vi "Draw Flatten Pixmap__jki_lib_picture -- VI Tester.vi"(10 "image data":T1, 11 "picture":picture) -> (3 "new picture":picture)   [LabVIEW 2011]
doc: "Draws a 1-, 4-, 8-bit pixmap, 24-bit RGB pixmap or a 32-bit ARGB pixmap into a picture. The transparency information in the 32-bit ARGB pixmap will be used to draw the pixmap over the existing picture.\n\n<B>Copyright © 2006 James Kring, Inc. All rights reserved.</B>\n\nAuthor: Philippe Guerit <<B>philippe.guerit@jameskring.com</B>>\n<alternate_email: <B>PJM_LabVIEW@yahoo.com</B>>\n\nThis library is provided \"AS IS\" , WITHOUT WARRANTIES OR \nCONDITIONS OF ANY KIND, either express or implied.\n\n<B>James Kring, Inc.</B> -- http://www.jameskring.com"
uses:
  <vilib>/picture/picture.llb/imagedata.ctl
panel:
  in  "Case Constant\n(See Context Help)":bool
  # "Copyright © 2006 James Kring, Inc. All rights reserved.\n\nAuthor: Philippe Guerit <philippe.guerit@jameskring.com>\n<alternate_email: PJM_LabVIEW@yahoo.com>\n\nThis library is provided \"AS IS\" , WITHOUT WARRANTIES OR \nCONDITIONS OF ANY KIND, either express or implied.\n\nJames Kring, Inc. -- http://www.jameskring.com"
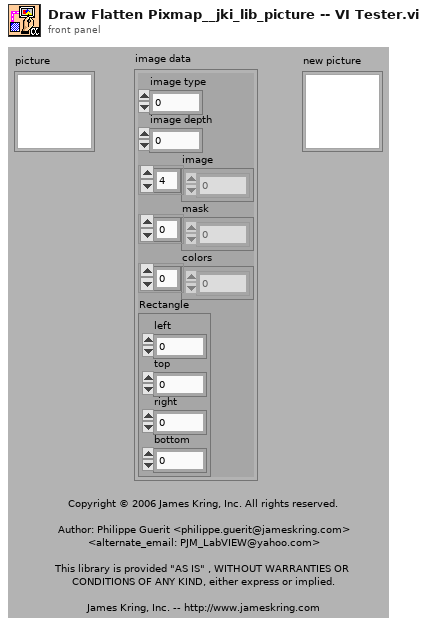
[diagram p1: front panel]
types:
  T1 = typedef "imagedata.ctl" = cluster{"image type":i32, "image depth":i32, "image":u8[], "mask":u8[], "colors":u32[], "Rectangle":cluster{"left":i16, "top":i16, "right":i16, "bottom":i16}}
  T2 = cluster{"left":i16, "top":i16, "right":i16, "bottom":i16}
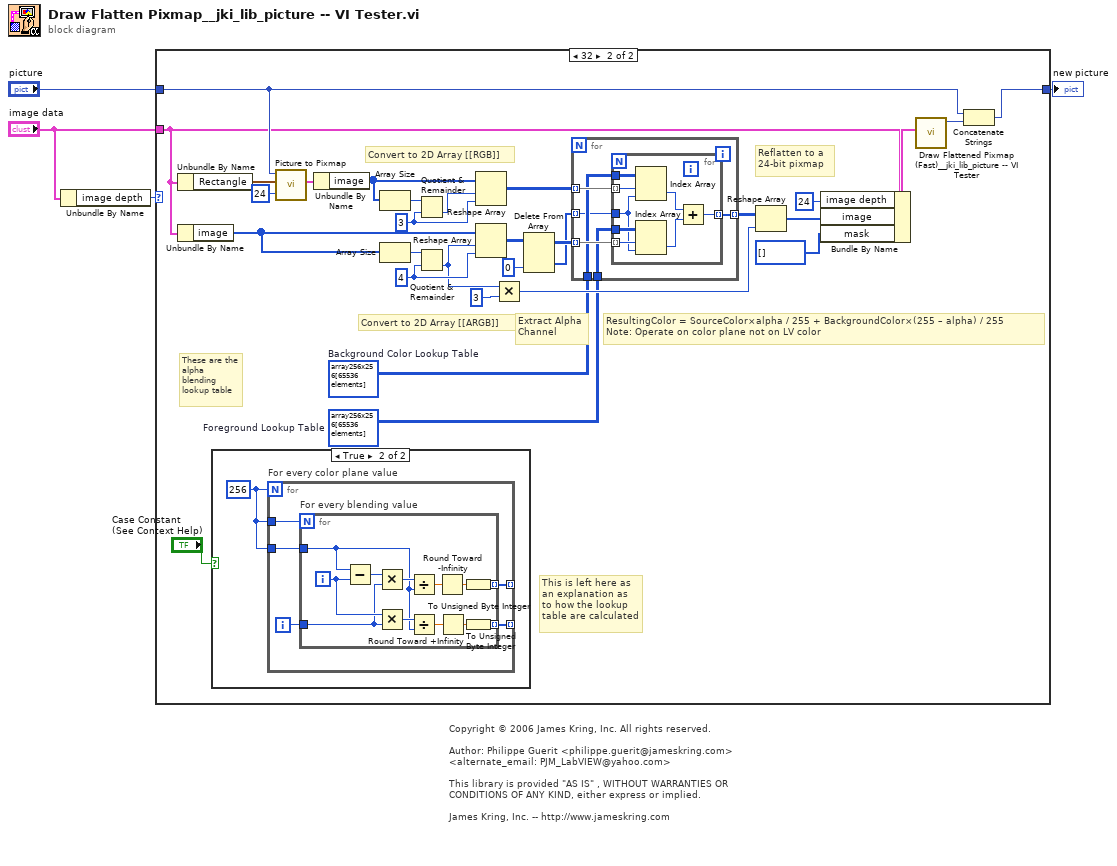
[diagram p0: block diagram]
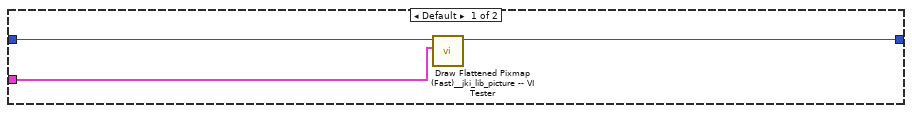
[diagram p2: hidden frame]
diagram:
  # "Copyright © 2006 James Kring, Inc. All rights reserved.\n\nAuthor: Philippe Guerit <philippe.guerit@jameskring.com>\n<alternate_email: PJM_LabVIEW@yahoo.com>\n\nThis library is provided \"AS IS\" , WITHOUT WARRANTIES OR \nCONDITIONS OF ANY KIND, either express or implied.\n\nJames Kring, Inc. -- http://www.jameskring.com"
  n1 = Unbundle By Name("image data") -> ("image depth"=w1:i32)
  n2 = case shown="32" w1 {
    tunnel: "image data" -> [w6 w12]
    tunnel: "picture" -> [w7 w18]
    tunnel: [w5 w19] -> w2
    frame Default {
      n3 = call "Draw Flattened Pixmap (Fast)__jki_lib_picture -- VI Tester.vi"("image data"=w6, "picture"=w7) -> ("new picture"=w5:picture)  [unwired: 7 in]
    }
    frame 32 {
      w9 = u8[][] array256x256[65536 elements]  # Foreground Lookup Table
      w10 = u8[][] array256x256[65536 elements]  # Background Color Lookup Table
      w30 = 3 ("y")
      w29 = 4 ("y")
      # "Reflatten to a 24-bit pixmap"
      # "Extract Alpha\nChannel"
      # "Convert to 2D Array [[ARGB]]"
      # "This is left here as an explanation as to how the lookup table are calculated"
      # "Convert to 2D Array [[RGB]]"
      # "These are the alpha blending lookup table"
      # "ResultingColor = SourceColor×alpha / 255 + BackgroundColor×(255 – alpha) / 255 \nNote: Operate on color plane not on LV color"
      n4 = Unbundle By Name(w12) -> ("Rectangle"=w37:T2)
      n5 = Unbundle By Name(w12) -> ("image"=w35:u8[])
      n6 = case shown="True" "Case Constant\n(See Context Help)" {
        frame False {
        }
        frame True {
          w38 = 256
          n7 = for "For every color plane value" {
            N: w38 -> [_]
            tunnel: w38 -> [w43]
            tunnel: w38 -> [w42]
            tunnel: [w40] -> _ mode=indexing
            tunnel: [w39] -> _ mode=indexing
            i -> [w41]
            n8 = for "For every blending value" {
              N: w43 -> [_]
              tunnel: w42 -> [w48]
              tunnel: w41 -> [w50]
              tunnel: [w53] -> w40 mode=indexing
              tunnel: [w46] -> w39 mode=indexing
              i -> [w52]
              n9 = Subtract(x=w48, y=w52) -> (x-y=w51:i32)
              n10 = Multiply(x=w51, y=w50) -> (x*y=w49:i32)
              n11 = Multiply(x=w52, y=w50) -> (x*y=w55:i32)
              n12 = Divide(x=w49, y=w48) -> (x/y=w47:dbl)
              n13 = Divide(x=w55, y=w48) -> (x/y=w54:dbl)
              n14 = Round Toward -Infinity(1:w47) -> (0:w45:dbl)
              n15 = Round Toward +Infinity(x=w54) -> (ceil(x): smallest int >= x=w44:dbl)
              n16 = To Unsigned Byte Integer(number=w45) -> (unsigned 8bit integer=w46:u8)
              n17 = To Unsigned Byte Integer(number=w44) -> (unsigned 8bit integer=w53:u8)
            }
          }
        }
      }
      n18 = call <vilib>:"Picture to Pixmap.vi"("depth"=24, "rect"=w37, "picture"=w18) -> ("image data"=w13:T1)  [unwired: 7 in, 1 out]
      n19 = Unbundle By Name(w13) -> ("image"=w31:u8[])
      n20 = Array Size(array=w31) -> (size(s)=w32:i32)
      n21 = Array Size(array=w35) -> (size(s)=w36:i32)
      n22 = Quotient & Remainder(x=w32, y=w30) -> (floor(x/y)=w22:i32)  [unwired: 1 out]
      n23 = Quotient & Remainder(x=w36, y=w29) -> (floor(x/y)=w26:i32)  [unwired: 1 out]
      n24 = Reshape Array(w31, w22, w30) -> (w14:u8[][])
      n25 = Reshape Array(w35, w26, w29) -> (w33:u8[][])
      n26 = Multiply(x=w26, y=3) -> (x*y=w25:i32)
      n27 = Delete From Array(array=w33, index (col)=0 ("dimension size")) -> (deleted portion=w15:u8[], array with subset deleted=w21:u8[][])  [unwired: 2 in]
      n28 = for {
        tunnel: w21 -> [w60] mode=indexing
        tunnel: w14 -> [w61] mode=indexing
        tunnel: w10 -> [w59]
        tunnel: w9 -> [w58]
        tunnel: [w56] -> w28 mode=indexing
        tunnel: w15 -> [w57] mode=indexing
        n29 = for {
          tunnel: w61 -> [w68] mode=indexing
          tunnel: w60 -> [w66] mode=indexing
          tunnel: w59 -> [w69]
          tunnel: w58 -> [w67]
          tunnel: [w63] -> w56 mode=indexing
          tunnel: w57 -> [w62]
          n30 = Index Array(array=w69, index (row)=w68, index (col)=w62) -> (element=w65:u8)
          n31 = Index Array(array=w67, index (row)=w66, index (col)=w62) -> (element=w64:u8)
          n32 = Add(x=w65, y=w64) -> (x+y=w63:u8)
        }
      }
      n33 = Reshape Array(w28, w25) -> (w11:u8[])
      n34 = Bundle By Name(cluster=w12, "image depth"=24, "image"=w11, "mask"=u8[] []) -> (w23:T1)
      n35 = call "Draw Flattened Pixmap (Fast)__jki_lib_picture -- VI Tester.vi"("image data"=w23) -> ("new picture"=w17:picture)  [unwired: 8 in]
      n36 = Concatenate Strings(w18, w17) -> (w19:picture)
    }
  }
  "new picture" <- w2
